vi "Write RT VI Properties.vi"(8 "Error In":errorcluster, 10 "Supported Targets Properties":T1, 11 "Custom Device .NET Ref In":refnum<k24>) -> (0 "Error Out":errorcluster, 3 "Custom Device .NET Ref Out":refnum<k24>)   [LabVIEW 2019, in "VeriStand Custom Device XML Parser.lvlib"]
doc: "Sets the properties for each supported target"
uses:
  VeriStand Custom Device XML Parser.lvlib
  NationalInstruments.VeriStand.XMLReader
  XML Controls/Custom Device Source Distribution Properties.ctl
  XML Controls/Path Cluster.ctl
  XML Controls/Supported Targets.ctl
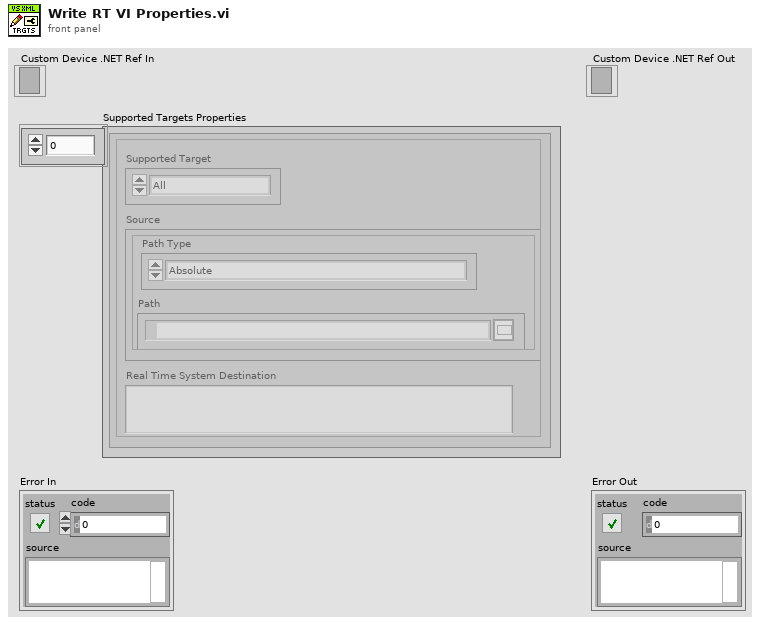
[diagram p1: front panel]
types:
  T1 = typedef "VeriStand Custom Device XML Parser.lvlib/Custom Device Source Distribution Properties.ctl" = cluster{"Source":T2, "Real Time System Destination":string, "Supported Target":T3}[]
  T2 = typedef "VeriStand Custom Device XML Parser.lvlib/Path Cluster.ctl" = cluster{"Path":path, "Path Type":enum16{"Absolute", "To Base", "To Common Doc Dir", "To Application Data Dir"}}
  T3 = typedef "VeriStand Custom Device XML Parser.lvlib/Supported Targets.ctl" = enum16{"All", "Pharlap", "VxWorks", "Windows", "Linux_32_ARM", "Linux_x64", "PharlapWindows", "PharlapVxWorks", "VxWorksWindows"}
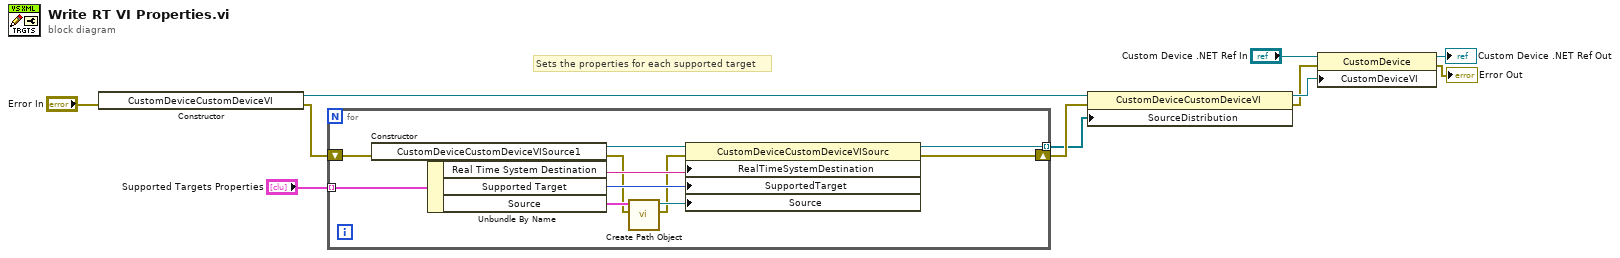
[diagram p0: block diagram]
diagram:
  # "Sets the properties for each supported target"
  n1 = constructor class="CustomDeviceCustomDeviceVI"(error in="Error In") -> (reference out=w5:refnum<k24>, error out=w4:errorcluster)  [unwired: 2 in, 1 out]
  n2 = for {
    shift-right: [w17] -> w7
    shift-left: w4 -> [w20]
    tunnel: "Supported Targets Properties" -> [w22] mode=indexing
    tunnel: [w16] -> w6 mode=indexing
    n3 = constructor class="CustomDeviceCustomDeviceVISourc"(error in=w20) -> (reference out=w21:refnum<k24>, error out=w14:errorcluster)  [unwired: 2 in, 1 out]
    n4 = Unbundle By Name(w22) -> ("Real Time System Destination"=w18:string, "Supported Target"=w19:T3, "Source"=w15:T2)
    n5 = call "Create Path Object.vi"("Error In"=w14, "Path Data Cluster"=w15) -> ("Error Out"=w12:errorcluster, "Path .NET Ref"=w13:refnum<k24>)  [unwired: 8 in]
    n6 = property class="CustomDeviceCustomDeviceVISourc"(reference=w21, error in=w12, "RealTimeSystemDestination"=w18, "SupportedTarget"=w19, "Source"=w13) -> (reference out=w16:refnum<k24>, error out=w17:errorcluster)
  }
  n7 = property class="CustomDeviceCustomDeviceVI"(reference=w5, error in=w7, "SourceDistribution"=w6) -> (reference out=w9:refnum<k24>, error out=w8:errorcluster)
  n8 = property class="CustomDevice"(reference="Custom Device .NET Ref In", error in=w8, "CustomDeviceVI"=w9) -> (reference out=→"Custom Device .NET Ref Out":refnum<k24>, error out=→"Error Out":errorcluster)
